vi "SteuerungWaermepumpe.vi"() -> ()   [LabVIEW 2015]
uses:
  <vilib>/DAQmx/read.llb/DAQmx Read (Analog 1D Wfm NChan NSamp).vi
  <vilib>/DAQmx/write.llb/DAQmx Write (Analog 1D Wfm NChan 1Samp).vi
  <vilib>/MakerHub/LINX/Public/Peripherals/Digital/Digital Write N Chans.vi
  <vilib>/DAQmx/miscellaneous.llb/DAQmx Fill In Error Info.vi
  <vilib>/Utility/file.llb/Read Delimited Spreadsheet (DBL).vi
  <vilib>/MakerHub/LINX/LMH-LINX.lvlib
panel:
  out "Abscheider":cluster{dbl, dbl, dbl}(slide) scale=0.0..1.3
  in  "Rampe":bool=TRUE
  in  "Rampe rpm/s":dbl=1.0 min=1.0 max=100.0 step=1.0
  out "Rampe IW":dbl
  in  "reinitialize HD":bool
  in  "reinitialize Pumpe":bool
  out "ist an!":string
  in  "zusätzlicher Druck":dbl
  in  "PI05 SW":dbl format="%.2f"
  out "p_liq_mittel":dbl
  out "p_liq":dbl
  out "Schleifendauer":dbl format="%.5f"
  out "Mittelwert 2":dbl
  in  "Mittelwert HD":bool
  in  "Mittelwert Pumpe":bool
  out "Mittelwert":dbl
  in  "Xi / p_liq berechnung an":bool
  out "xi_r":dbl
  in  "Regler Senke":bool
  in  "reinitialize Senke":bool
  in  "TI35 SW":dbl=43.0 format="%.2f"
  in  "Drehzahl Bestätigung":bool
  in  "Drehzahl SW":dbl=1000.0 min=500.0 max=3000.0 step=1.0 format="%#_4g"
  out "Check":dbl format="%#_13g"
  in  "Regler Hochdruck":bool
  in  "PID Regelung Pumpe":bool
  in  "SW TI39":dbl
  out "Array":bool[](array[boolean])
  in  "LEDs 2":bool[](array[boolean])
  in  "Regelung HK":bool
  in  "zu":bool
  in  "auf":bool
  out "FI_Oel":dbl
  in  "RV 33":dbl(slide) scale=-1.0..1.0
  in  "tag":string
  out "Pumpenwerte":dbl[](array[numeric]) format="%.2f"
  out "Speichert!":bool
  out "Historie":string
  in  "Kommentar":string
  out "refnum out":refnum<file>
  in  "Identität!":string(combo)
  in  "Zeit X in Minuten":dbl(slide)=5.0 min=0.0 max=15.0 scale=5.0..15.0
  out "TI 21a Warnungen":dbl
  out "Leistung":dynamicdata(graph)
  out "TI 37":dbl
  in  "Programm stoppen!":bool
  out "%":sgl(slide) scale=0.0..100.0
  out "kalt":bool
  out "warm":bool
  out "?":T1(array[cluster]) {"?" format="%#.4g"; "Konzentration_reich" format="%#.4g"}
  in  "Mit EES vergleichen":bool
  in  "FI13 SW in l/min":dbl=3.0 min=3.0 max=12.0 step=0.10000000149011612
  out "COP_Oel":dbl
  out "Q-Oel kW":dbl format="%_4g"
  in  "Dateiname!":string
  in  "Comment":bool
  in  "Speichern":bool caption="Aktivieren"
  out "ZU     Ventilstellung 33     AUF":dbl(slide) scale=0.0..100.0 scale format="%.2f"
  in  "Regelventil 34":dbl(slide) min=0.0 max=100.0 step=0.009999999776482582 scale=0.0..100.0
  in  "Matlab":bool
  in  "?":T2(tab)
  out "?":dynamicdata(graph)
  out "?":waveform(dbl)(graph)
  out "?":dynamicdata(graph)
  out "PI 12":dbl format="%.2f"
  out "PI 11":dbl format="%.2f"
  out "Dichte":dbl format="%.5g"
  in  "Reset":bool
  out "Betriebszeit":cluster{"second":i32, "minute":i32, "hour":i32}
  out "Temperatur Ölprüfstand":dbl
  out "FI 13 kg/min":dbl
  in  "Messung\nFrequenzwandler":bool
  out "Magnetventil":bool
  out "Fl.Pumpe an":bool
  out "Temperatur Öl":bool
  out "COP":dbl format="%#_13g"
  out "Verdichteraktivität":cluster{"second":i32, "minute":i32, "hour":i32}
  out "Q-Entgaser kW":dbl format="%_4g"
  out "Warnungen":bool[](array[boolean])
  out "Status Komponenten":bool[](array[boolean])
  in  "Pumpen-Auto-Abschalt":bool=TRUE
  out "Q-Resorber kW":dbl format="%_4g"
  out "Stellung Expansionsventil":waveform(dbl)(graph)
  out "FI 35 l/min":dbl format="%#_13g"
  out "FI 38 l/min":dbl format="%#_13g"
  out "FI Oel l/min":dbl format="%#.3g"
  out "LI in l":dbl format="%#_4g"
  out "TI 39":dbl format="%#_3g"
  out "TI 38":dbl format="%#_3g"
  out "TI 36":dbl format="%#_3g"
  out "TI 35":dbl format="%#_3g"
  out "TI 33":dbl format="%#_3g"
  out "TI 32":dbl format="%#_3g"
  out "TI 34":dbl format="%#_3g"
  out "TI 21a":dbl format="%#_3g"
  out "TI 21":dbl format="%#_3g"
  out "TI 20":dbl format="%#_3g"
  out "TI 14a":dbl format="%#_3g"
  out "TI 14":dbl format="%#_3g"
  out "TI 13":dbl format="%#_3g"
  out "TI 12":dbl format="%#_3g"
  out "TI 11":dbl format="%#_3g"
  out "TI 10":dbl format="%#_3g"
  out "TI 09":dbl format="%#_3g"
  out "TI 08":dbl format="%#_3g"
  out "TI 07":dbl format="%#_3g"
  out "TI 06a":dbl format="%#_3g"
  out "TI 06":dbl format="%#_3g"
  out "TI 05":dbl format="%#_3g"
  out "TI 04":dbl format="%#_3g"
  out "TI 22":dbl format="%#_3g"
  out "TI 02":dbl format="%#_3g"
  out "TI 01":dbl format="%#_3g"
  out "Konzentration":dbl format="%#_5g"
  in  "Pumpensteuerung":dbl min=0.0 max=10.0 step=0.009999999776482582 format="%.2g"
  out "PI 08":dbl format="%.2f"
  out "PI 05":dbl format="%#.2f"
  out "PI 02":dbl format="%.2f"
  out "PI 04":dbl format="%.2f"
  out "PDI 8-9":dbl format="%.2f"
  out "PI 14":dbl format="%.2f"
  out "PI 01":dbl format="%.2f"
  out "ZU    Ventilstellung Exp.V     AUF":dbl(slide) scale=0.0..100.0 scale format="%#.1f"
  in  "Exp.V":dbl(slide)=3.0 min=0.0 max=100.0 step=1.0 scale=0.0..100.0 scale format="%#.0f"
  out "ZU    Ventilstellung 14      AUF":dbl(slide) caption="Auf    Ventilstellung 14      Zu" scale=0.0..100.0 scale format="%#.2f"
  in  "Regelventil 36":dbl(slide) min=0.0 max=100.0 step=0.009999999776482582 scale=0.0..100.0 scale format="%#.0f"
  out "ZU  Ventilstellung 35  AUF":dbl(slide) scale=0.0..100.0 scale format="%.2f"
  in  "Regelventil 35":dbl(slide)=100.0 min=0.0 max=100.0 step=0.009999999776482582 scale=0.0..100.0 scale format="%#.3g"
  out "ZU     Ventilstellung 39     AUF":dbl(slide) scale=0.0..100.0 scale format="%.2f"
  in  "Regelventil 39":dbl(slide)=100.0 min=0.0 max=100.0 step=0.009999999776482582 scale=0.0..100.0
  out "FI 13 l/min":dbl format="%.2f"
  out "FI 07 l/min":dbl format="%.2f"
  out "LI in m":dbl format="%.2f"
  out "PDI 5-6":dbl format="%.4f"
  out "PI 07":dbl format="%.2f"
  out "Druckverhältnis":dbl
  out "Drehzahl":dbl
  out "Drehmoment":dbl
  out "Frequenz":dbl
  out "Leistung":dbl
  out "Durchfluss":waveform(dbl)[](graph)
  in  "Tab Control Temperaturen":T3(tab)
  out "Temperatur Reich":waveform(dbl)[](graph)
  out "Temperatur Arm":waveform(dbl)[](graph)
  out "Temperatur Öl":waveform(dbl)[](graph)
  out "Temperatur Senke/Quelle":waveform(dbl)[](graph)
  out "Druck":waveform(dbl)[](graph)
  out "Druckzustand":bool caption="Zu viel Druck !!!"
  # "Öltemperatur"
  # "Resorber"
  # "Entgaser"
  # "Druckverhältnis"
  # "ExpV"
  # "Verdichter an"
  # "iWÜ"
  # "Magnetventil"
  # "RV 39"
  # "RV 35"
  # "RV 33"
  # "RV 34"
  # "Pumpe an"
  # "Ölabscheider"
  # "2"
  # "1"
  # "RV 30"
  # "Verdichter"
  # "Pumpe"
  # "Leistung"
  # "kW"
  # "Speed"
  # "rpm"
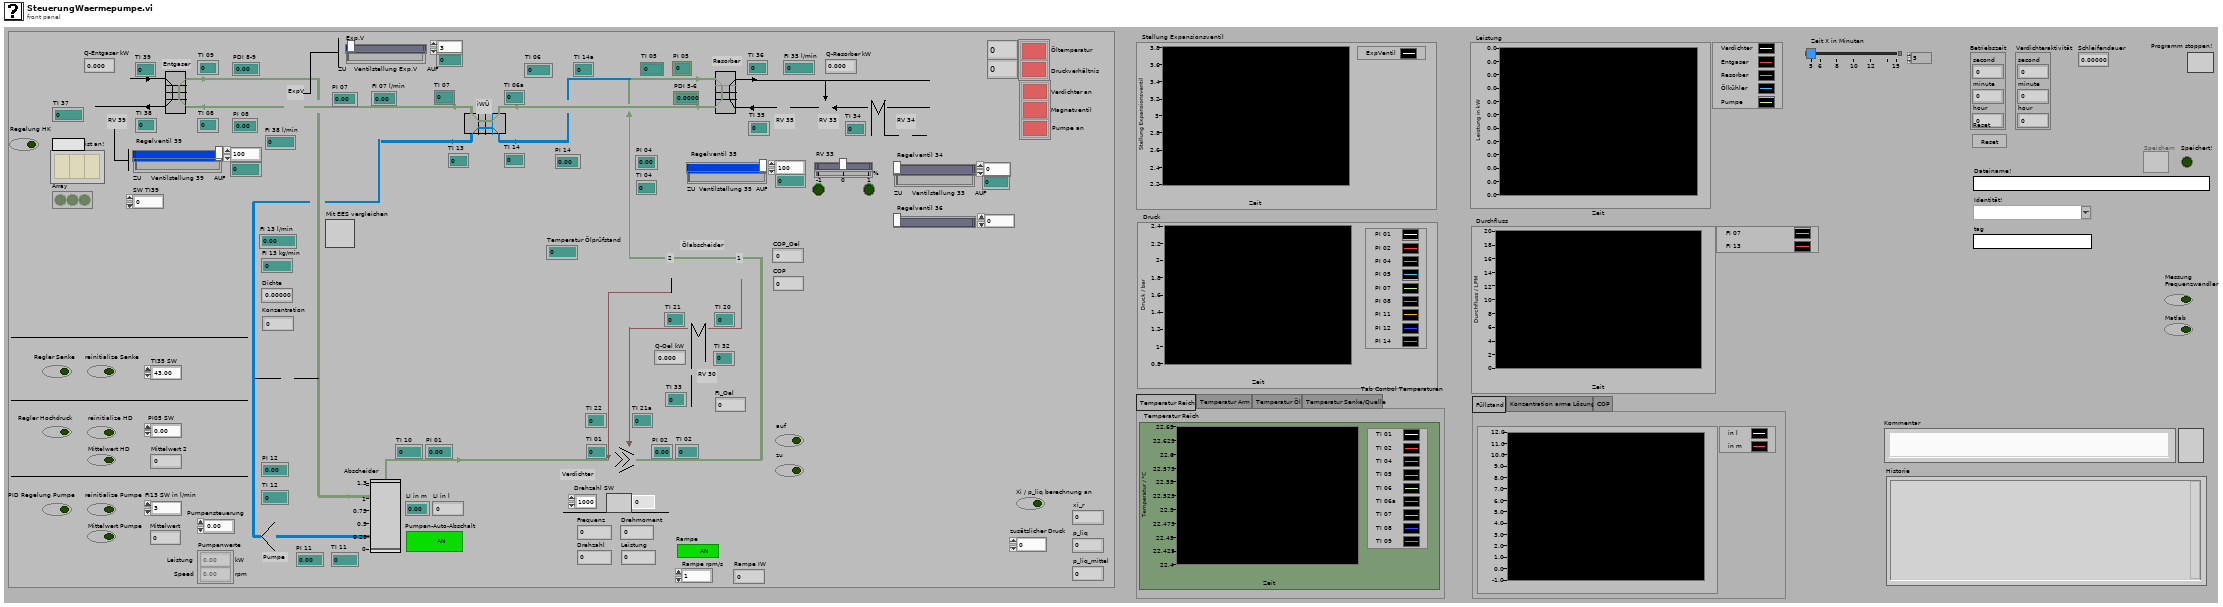
[diagram p1: front panel]
types:
  T1 = cluster{dbl, "Konzentration_reich":dbl, "String":string, bool}[]
  T2 = enum32{"Füllstand", "Konzentration arme Lösung", "COP"}
  T3 = enum32{"Temperatur Reich", "Temperatur Arm", "Temperatur Öl", "Temperatur Senke/Quelle"}
  T4 = enum8{"Enabled", "Disabled", "Disabled and Grayed Out"}
  T5 = typedef "LMH-LINX.lvlib/LINX Ref.ctl" = cluster{"Platform":T6, "Interface":T7, "LINX Device Config":T8}
  T6 = typedef "LMH-LINX.lvlib/Platform.ctl" = enum16{"LINX", "myRIO"}
  T7 = typedef "LMH-LINX.lvlib/Interface.ctl" = enum16{"Serial", "TCP"}
  T8 = typedef "LMH-LINX.lvlib/Device.lvlib/LINX Device Config.ctl" = cluster{"Interface":T7, "COM Port":refnum<visa-resource-name>, "TCP Configuration":T9, "Device Family":u8, "Device ID":u8, "Device Name":string, "TCP Ref":refnum<k5>, "Channels":T10}
  T9 = typedef "LMH-LINX.lvlib/Device.lvlib/TCP Config.ctl" = cluster{"IP Address":string, "Port":u16}
  T10 = typedef "LMH-LINX.lvlib/Channels.ctl" = cluster{"DI":u8[], "DO":u8[], "AI":u8[], "AO":u8[], "PWM":u8[], "QE":u8[], "UART":u8[], "I2C 2":u8[], "SPI":u8[], "CAN":u8[], "Servo":u8[], "AI Ref (V)":dbl, "AO Ref (V)":dbl, "AO Resolution (Bits)":u8}
  T11 = enum16{"open", "replace", "create", "open or create", "replace or create", "replace or create with confirmation"}
  T12 = cluster{"Array[0]":dbl, "Array[1]":dbl, "Array[2]":dbl}
  T13 = cluster{"Array[0]":sgl, "Array[1]":sgl, "Array[2]":sgl}
  T14 = cluster{"Numeric":dbl, "Konzentration_reich":dbl, "String":string, bool}[]
  T15 = typedef "LVDateTimeRec.ctl" = cluster{"fractional second":dbl, "second":i32, "minute":i32, "hour":i32, "day of month":i32, "month":i32, "year":i32, "day of week":i32, "day of year":i32, "DST":i32}
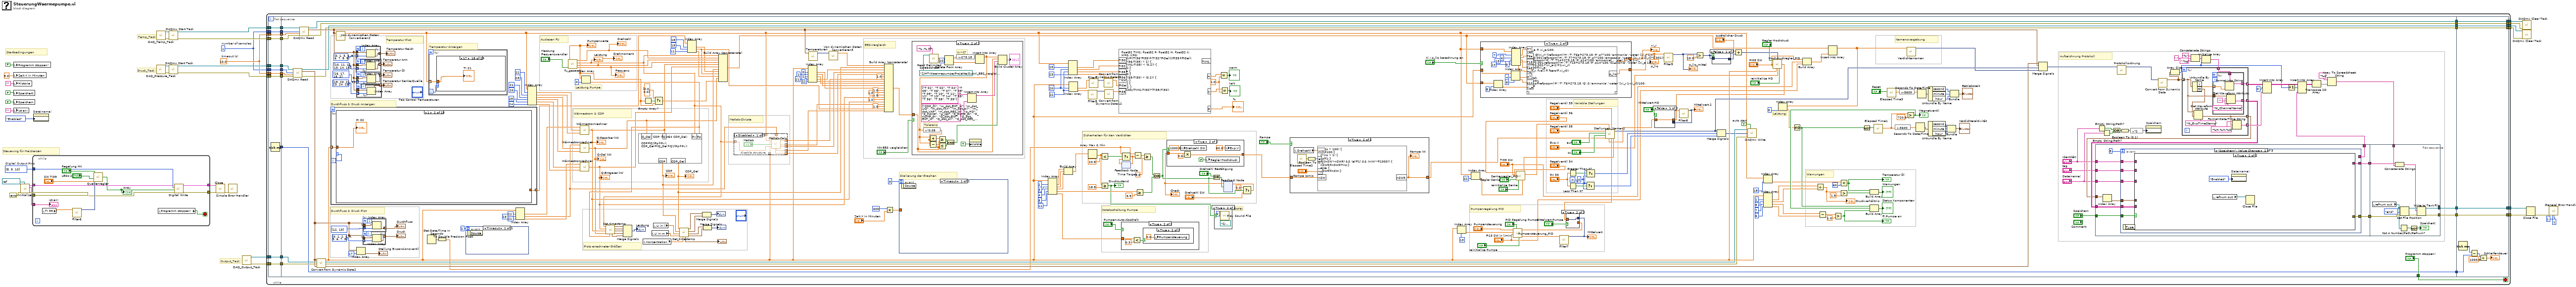
[diagram p0: block diagram]
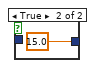
[diagram p5: hidden frame]
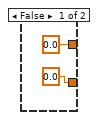
[diagram p8: hidden frame]
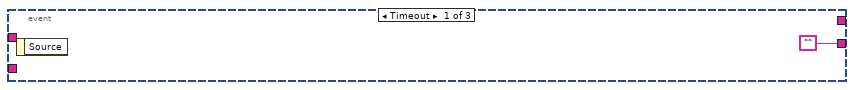
[diagram p10: hidden frame]
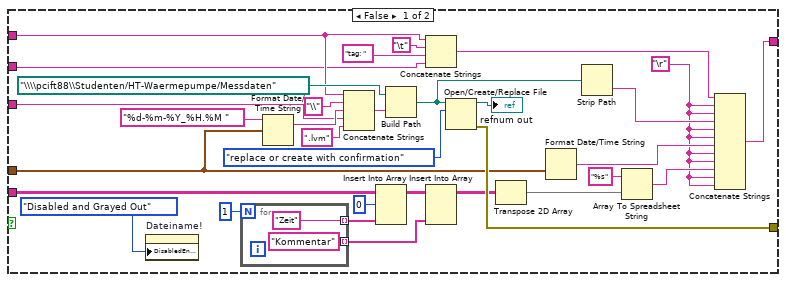
[diagram p11: hidden frame]
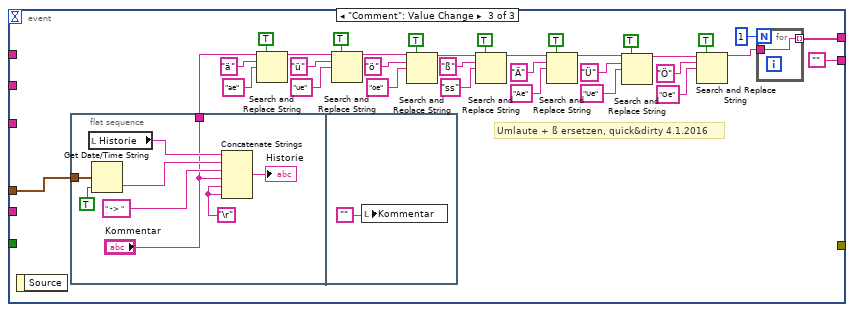
[diagram p12: hidden frame]
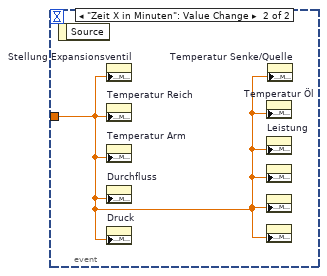
[diagram p13: hidden frame]
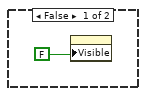
[diagram p14: hidden frame]
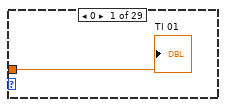
[diagram p17: hidden frame]
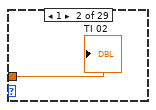
[diagram p18: hidden frame]
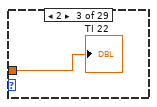
[diagram p19: hidden frame]
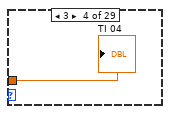
[diagram p20: hidden frame]
diagram:
  w9 = 10.0  # timeout (s)
  w8 = 1  # number of samples
  w21 = i32[] [8, 9, 10]  # Digital Output PIns
  # "Output_Task"
  # "Druck_Task"
  # "Temp_Task"
  # "Steuerung für Heizkerzen"
  # "Startbedingungen"
  n1 = local write "Programm stoppen!"(FALSE ("Programm stoppen!")) -> ()
  n2 = local write "Zeit X in Minuten"(5.0 ("Zeit X in Minuten")) -> ()
  n3 = local write "Historie"("") -> ()
  n4 = local write "Speichert!"(FALSE ("Speichert!")) -> ()
  n5 = local write "Speichern"(FALSE ("Speichern")) -> ()
  n6 = local write "ist an!"("") -> ()
  n7 = call <vilib>:"Initialize.vi"("Serial Port"=refnum<visa-resource-name> "COM3", "Error In"=errorcluster {"status"=FALSE, "code"=0, "source"=""}) -> ("Error Out"=w22:errorcluster, "Device Name"=w19:string, "LINX Ref"=w25:T5)  [unwired: 7 in]
  n8 = while {
    tunnel: w25 -> [w40]
    tunnel: [w50] -> w24
    tunnel: [w49] -> w23
    tunnel: w22 -> [w39]
    tunnel: w21 -> [w48]
    tunnel: w19 -> [w38]
    stop <- w47 stop-if-true
    n9 = local read "TI 39"() -> (w41:dbl)
    n10 = call "Filter6"("Signal"=w41) -> ("Filtered Signal"=w42:dynamicdata)  [unwired: 9 in, 1 out]
    n11 = call "Quellenregler.vi"("Regelung Quelle"="Regelung HK", "TI 38 IW °C"=w42, "LEDs"="LEDs 2", "TI 38 SW °C"="SW TI39") -> ("Kerzen von Regler"=w44:bool[])  [unwired: 3 in, 1 out]
    "Array" <- w44
    n12 = local read "Programm stoppen!"() -> (w47:bool)
    n13 = call-poly <vilib>:"Digital Write.vi"("Error In"=w39, "Values"=w44, "DO Channels"=w48, "LINX Resource"=w40) -> ("Error Out"=w49:errorcluster, "LINX Resource"=w50:T5)  [unwired: 6 in]
    "ist an!" <- w38
  }
  n14 = property on="Dateiname!" class="Str"("DisabledEnum"=T4."Enabled" ("Disabled")) -> ()  [unwired: 2 in, 2 out]
  n15 = call "DAQ_Pressure_Task.vi"() -> ("error out"=w13:errorcluster, "task out"=w14:refnum<k21>)  [unwired: 10 in]
  n16 = call "DAQ_Temp_Task.vi"() -> ("error out"=w15:errorcluster, "task out"=w16:refnum<k21>)  [unwired: 10 in]
  n17 = call <vilib>:"DAQmx Start Task.vi"("task/channels in"=w14, "error in"=w13) -> ("task out"=w7:refnum<k21>, "error out"=w10:errorcluster)  [unwired: 12 in]
  n18 = call <vilib>:"DAQmx Start Task.vi"("task/channels in"=w16, "error in"=w15) -> ("task out"=w11:refnum<k21>, "error out"=w12:errorcluster)  [unwired: 12 in]
  n19 = call <vilib>:"Close.vi"("Error In"=w23, "LINX Resource"=w24) -> ("Error Out"=w26:errorcluster)  [unwired: 8 in, 1 out]
  n20 = call <vilib>:"Simple Error Handler.vi"("error in (no error)"=w26) -> ()  [unwired: 4 in, 5 out]
  n21 = call "DAQ_Output_Task.vi"() -> ("error out"=w1:errorcluster, "task out"=w2:refnum<k21>)  [unwired: 10 in]
  n22 = while {
    tunnel: [w85] -> w31
    tunnel: [w84] -> w30
    tunnel: w12 -> [w78]
    tunnel: w9 -> [w76]
    tunnel: w11 -> [w73]
    tunnel: w8 -> [w71]
    tunnel: w10 -> [w69]
    tunnel: w9 -> [w68]
    tunnel: w8 -> [w66]
    tunnel: w7 -> [w64]
    tunnel: [w60] -> w6
    tunnel: [w59] -> w5
    tunnel: [w57] -> w4
    tunnel: [w55] -> w3
    tunnel: w2 -> [w54]
    tunnel: w1 -> [w51]
    stop <- w83 stop-if-true
    n23 = flat-sequence {
      tunnel: [w96] -> w79
      tunnel: w78 -> [w95]
      tunnel: [w95] -> w77
      tunnel: w76 -> [w94]
      tunnel: [w94] -> w75
      tunnel: w73 -> [w93]
      tunnel: [w93] -> w74
      tunnel: [w92] -> w72
      tunnel: w71 -> [w92]
      tunnel: [w91] -> w70
      tunnel: w69 -> [w91]
      tunnel: w68 -> [w90]
      tunnel: [w90] -> w67
      tunnel: w66 -> [w89]
      tunnel: [w89] -> w65
      tunnel: w64 -> [w88]
      tunnel: [w88] -> w63
      tunnel: w54 -> [w87]
      tunnel: [w87] -> w53
      tunnel: [w86] -> w52
      tunnel: w51 -> [w86]
      tunnel: ["Programm stoppen!"] -> w83
      tunnel: [w304] -> w82
      tunnel: [w303] -> w81
      tunnel: [w102] -> w80
      tunnel: w79 -> [w102]
      tunnel: w77 -> [w143]
      tunnel: w75 -> [w142]
      tunnel: w74 -> [w141]
      tunnel: w72 -> [w140]
      tunnel: w70 -> [w139]
      tunnel: w67 -> [w138]
      tunnel: w65 -> [w137]
      tunnel: w63 -> [w136]
      tunnel: [w135] -> w62
      tunnel: [w134] -> w61
      tunnel: [w133] -> w58
      tunnel: [w132] -> w56
      tunnel: w53 -> [w130]
      tunnel: w52 -> [w129]
      tunnel: [w722] -> w84
      tunnel: [w723] -> w85
      tunnel: w82 -> [w723]
      tunnel: w81 -> [w722]
      tunnel: w80 -> [w720]
      tunnel: w62 -> [w715]
      tunnel: w61 -> [w716]
      tunnel: [w716] -> w60
      tunnel: [w715] -> w59
      tunnel: w58 -> [w714]
      tunnel: [w714] -> w57
      tunnel: w56 -> [w713]
      tunnel: [w713] -> w55
      frame #0 {
        n24 = Tick Count (ms)() -> (millisecond timer value=w96:u32)
      }
      frame #1 {
        w104 = 8.0  # Time Target
        w131 = TRUE  # auto start
        w324 = sgl 1.0
        w337 = 22
        w342 = 20
        w368 = -4
        w369 = 0
        # "ENTE!"
        # "Sicherheiten für den Verdichter"
        # "Pumpenregelung PID"
        # "Skalierung der Graphen"
        # "Leistung Pumpe"
        # "Leistung"
        # "Durchfluss & Druck Anzeigen"
        # "Temperatur Anzeigen"
        # "Plots errechneter Größen"
        # "EES-Vergleich"
        # "Matlab-Skripte"
        # "Warnungen"
        # "Namensvergebung"
        # "Wärmestrom & COP"
        # "Notabschaltung Pumpe"
        # "Auslesen FU"
        # "Durchfluss & Druck Plot"
        # "Temperatur Plot"
        # "Aufzeichnung Protokoll"
        # "Variable Stellungen"
        n25 = call-poly <vilib>:"DAQmx Read.vi"("task/channels in"=w136, "number of samples per channel"=w137, "timeout"=w138, "error in"=w139) -> ("task out"=w135:refnum<k21>, "data"=w145:waveform(dbl)[], "error out"=w132:errorcluster)  [unwired: 9 in]
        n26 = call-poly <vilib>:"DAQmx Read.vi"("task/channels in"=w141, "number of samples per channel"=w140, "timeout"=w142, "error in"=w143) -> ("task out"=w134:refnum<k21>, "data"=w144:waveform(dbl)[], "error out"=w133:errorcluster)  [unwired: 9 in]
        n27 = call "Convert from Dynamic Data2"("Dynamic Data Type"=w145) -> ("Array"=w150:dbl[])  [unwired: 3 in]
        n28 = for {
          tunnel: w150 -> [w661] mode=indexing
          tunnel: [w660] -> w155 mode=indexing
          i -> [w662]
          n29 = case shown="1" w662 {
            tunnel: w661 -> [w663 w664 w665 w666 w667 w668 w669 w670 w671 w672 w673 w682 w694 w697 w698 w699 w700 w701 w704 w708 w709 w710 w711 w712 _]
            tunnel: [_ _ _ _ _ _ _ _ _ _ _ w674 _ _ _ _ _ _ w702 w706 _ _ _ _ _] -> w660
            frame 0 {
              "PI 01" <- w663
            }
            frame 1 {
              "PI 02" <- w664
            }
            frame 2 {
              "PI 04" <- w665
            }
            frame 3 {
              "PI 05" <- w666
            }
            frame 4 {
              "PI 07" <- w667
            }
            frame 5 {
              "PI 08" <- w668
            }
            frame 6 {
              "PI 11" <- w669
            }
            frame 7 {
              "PI 12" <- w670
            }
            frame 8 {
              "PI 14" <- w671
            }
            frame 9 {
              "PDI 5-6" <- w672
            }
            frame 10 {
              "PDI 8-9" <- w673
            }
            frame 11 {
              n30 = call "Filter3"("Signal"=w682) -> ("Filtered Signal"=w680:dynamicdata)  [unwired: 9 in, 1 out]
              n31 = Greater?(x=w682, y=0.3) -> (0:w677:bool)
              n32 = case shown="False" w677 {
                tunnel: w682 -> [_ w693]
                tunnel: [0.0 w693] -> w685
                frame False {
                }
                frame True {
                }
              }
              n33 = call "Convert from Dynamic Data6"("Dynamic Data Type"=w680) -> ("Scalar"=w679:dbl)  [unwired: 3 in]
              n34 = Multiply(x=w679, y=10.0) -> (x*y=w681:dbl)
              n35 = Greater?(x=w682, y=0.4) -> (0:w678:bool)
              n36 = formula code="float64 y; float64 Vu; /*Vu: Volumen schmaler Zylinder+Fuellstandsmesser*/\nVu=10;  /* 10 Liter */\n\nif (x<=10.25) \ny=(x-1)*pi*(0.536**2+0.32**2);\nelse\ny=Vu+(x-10.25)*pi*(1.584**2+0.32**2);"("x"=w681) -> ("y"=w674:dbl)
              "LI in l" <- w674
              n37 = case shown="False" w678 {
                tunnel: w682 -> [_ w691]
                tunnel: [0.0 w691] -> w684
                frame False {
                }
                frame True {
                }
              }
              n38 = Merge Signals(w682, w685, w684) -> (w686:dynamicdata)
              n39 = call "Convert from Dynamic Data3"("Dynamic Data Type"=w686) -> ("Array"=w689:dbl[])  [unwired: 3 in]
              n40 = Array To Cluster(array=w689) -> (cluster=w676:T12)
              n41 = To Single Precision Float(number=w676) -> (single precision float=→"Abscheider":T13)
              "LI in m" <- w682
            }
            frame 12 {
              "FI 07 l/min" <- w694
            }
            frame 13 {
              n42 = local read "Dichte"() -> (w696:dbl)
              n43 = Multiply(x=w697, y=w696) -> (x*y=→"FI 13 kg/min":dbl)
              "FI 13 l/min" <- w697
            }
            frame 14 {
              "ZU     Ventilstellung 39     AUF" <- w698
              "ZU     Ventilstellung 33     AUF" <- w698
            }
            frame 15 {
              "ZU  Ventilstellung 35  AUF" <- w699
            }
            frame 16 {
              # "RV14 ist entfernt"
              "ZU    Ventilstellung 14      AUF" <- w700
            }
            frame 17 {
              "ZU    Ventilstellung Exp.V     AUF" <- w701
            }
            frame 18 {
              n44 = call "Filter"("Signal"=w704) -> ("Filtered Signal"=w703:dynamicdata)  [unwired: 9 in, 1 out]
              n45 = call "Convert from Dynamic Data4"("Dynamic Data Type"=w703) -> ("Scalar"=w705:dbl)  [unwired: 3 in]
              n46 = formula code="float64 D;\nD=9.375*StromDichte+0.7125;\nD=floor(D*100000)/100000;"("StromDichte"=w705) -> ("D"=w702:dbl)
              "Dichte" <- w702
            }
            frame 19 {
              n47 = call "Filter2"("Signal"=w708) -> ("Filtered Signal"=w707:dynamicdata)  [unwired: 9 in, 1 out]
              n48 = To Double Precision Float(number=w707) -> (double precision float=w706:dbl)
              "Konzentration" <- w706
            }
            frame 20 {
              "FI Oel l/min" <- w709
            }
            frame 21 {
              "FI 38 l/min" <- w710
            }
            frame 22 {
              "FI 35 l/min" <- w711
            }
            frame 23 {
              "FI_Oel" <- w712
            }
            frame 24, Default {
            }
          }
        }
        n49 = call "Von dynamischen Daten konvertieren2"("Dynamic Data Type"=w144) -> ("Array"=w125:dbl[])  [unwired: 3 in]
        n50 = for {
          tunnel: i32[] [0, 1, 3, 4, 5, 6, 7, 8, 9] -> [w475] mode=indexing
          tunnel: w144 -> [w474]
          tunnel: [w473] -> w240 mode=indexing
          n51 = Index Array(array=w474, index=w475) -> (element=w473:waveform(dbl))
        }
        "Temperatur Reich" <- w240
        n52 = for {
          tunnel: i32[] [10, 11, 12, 13, 14, 15] -> [w472] mode=indexing
          tunnel: w144 -> [w471]
          tunnel: [w470] -> w241 mode=indexing
          n53 = Index Array(array=w471, index=w472) -> (element=w470:waveform(dbl))
        }
        "Temperatur Arm" <- w241
        n54 = for {
          tunnel: i32[] [16, 17, 18, 2] -> [w469] mode=indexing
          tunnel: w144 -> [w468]
          tunnel: [w467] -> w242 mode=indexing
          n55 = Index Array(array=w468, index=w469) -> (element=w467:waveform(dbl))
        }
        "Temperatur Öl" <- w242
        n56 = Index Array(array=w145, index=17) -> (element=→"Stellung Expansionsventil":waveform(dbl))
        n57 = for {
          tunnel: i32[] [19, 20, 21, 22, 23, 24, 25] -> [w466] mode=indexing
          tunnel: w144 -> [w465]
          tunnel: [w464] -> w243 mode=indexing
          n58 = Index Array(array=w465, index=w466) -> (element=w464:waveform(dbl))
        }
        "Temperatur Senke/Quelle" <- w243
        n59 = for {
          tunnel: [w460] -> w238 mode=indexing
          tunnel: w145 -> [w459]
          tunnel: i32[] [0, 1, 2, 3, 4, 5, 6, 7, 8] -> [w458] mode=indexing
          n60 = Index Array(array=w459, index=w458) -> (element=w460:waveform(dbl))
        }
        "Druck" <- w238
        n61 = for {
          tunnel: [w463] -> w239 mode=indexing
          tunnel: w145 -> [w462]
          tunnel: i32[] [12, 13] -> [w461] mode=indexing
          n62 = Index Array(array=w462, index=w461) -> (element=w463:waveform(dbl))
        }
        "Durchfluss" <- w239
        n63 = Get Date/Time In Seconds() -> (seconds since 1Jan1904=w101:timestamp)
        n64 = for {
          tunnel: w125 -> [w630] mode=indexing
          i -> [w631]
          n65 = case shown="17" w631 {
            tunnel: w630 -> [w632 w633 w634 w635 w636 w637 w638 w639 w640 w641 w642 w643 w644 w645 w646 w647 w648 w649 w650 w651 w652 w653 w654 w655 w656 w657 w658 w659 _]
            frame 0 {
              "TI 01" <- w632
            }
            frame 1 {
              "TI 02" <- w633
            }
            frame 2 {
              "TI 22" <- w634
            }
            frame 3 {
              "TI 04" <- w635
            }
            frame 4 {
              "TI 05" <- w636
            }
            frame 5 {
              "TI 06" <- w637
            }
            frame 6 {
              "TI 06a" <- w638
            }
            frame 7 {
              "TI 07" <- w639
            }
            frame 8 {
              "TI 08" <- w640
            }
            frame 9 {
              "TI 09" <- w641
            }
            frame 10 {
              "TI 10" <- w642
            }
            frame 11 {
              "TI 11" <- w643
            }
            frame 12 {
              "TI 12" <- w644
            }
            frame 13 {
              "TI 13" <- w645
            }
            frame 14 {
              "TI 14" <- w646
            }
            frame 15 {
              "TI 14a" <- w647
            }
            frame 16 {
              "TI 20" <- w648
            }
            frame 17 {
              "TI 21" <- w649
            }
            frame 18 {
              "TI 21a" <- w650
              "TI 21a Warnungen" <- w650
            }
            frame 19 {
              # "Check T_Heater"
              "TI 34" <- w651
            }
            frame 20 {
              "TI 32" <- w652
            }
            frame 21 {
              "TI 33" <- w653
            }
            frame 22 {
              "TI 35" <- w654
            }
            frame 23 {
              "TI 36" <- w655
            }
            frame 24 {
              "TI 38" <- w656
            }
            frame 25 {
              "TI 39" <- w657
            }
            frame 26 {
              "Temperatur Ölprüfstand" <- w658
            }
            frame 27 {
              "TI 37" <- w659
            }
            frame 28, Default {
            }
          }
        }
        n66 = To Double Precision Float(number=w101) -> (double precision float=w100:dbl)
        n67 = event shown="[0] Timeout" {
          selector: _ -> [_]
          dyn-events: _ -> [_]
          timeout: 2 -> [_]
          event Timeout {
            n68 = event-data() -> ()  [unwired: 1 in, 1 out]
          }
        }
        n69 = Index Array(array=w150, index #1=22 ("index"), index #2=23 ("index"), index #3=21 ("index")) -> (element #1=w273:dbl, element #2=w249:dbl, element #3=w272:dbl)
        n70 = Index Array(array=w125, index #1=22 ("index"), index #2=23 ("index"), index #3=21 ("index"), index #4=20 ("index"), index #5=25 ("index"), index #6=24 ("index")) -> (element #1=w271:dbl, element #2=w270:dbl, element #3=w269:dbl, element #4=w268:dbl, element #5=w267:dbl, element #6=w266:dbl)
        n71 = call "fu_gesamt.vi"("Boolean"="Messung\nFrequenzwandler") -> ("Frequenz"=w261:dbl, "Drehmoment"=w262:dbl, "Leistung"=w113:dbl, "Drehzahl"=w263:dbl, "Scaled"=w115:dbl[])  [unwired: 6 in]
        "Leistung" <- w113
        "Frequenz" <- w261
        "Drehmoment" <- w262
        "Drehzahl" <- w263
        "Pumpenwerte" <- w115
        n72 = call "Wärmestromrechner.vi"("Taus"=w270, "Tein"=w271, "Massenstrom"=w273) -> ("Wärmestrom Q"=w169:dbl)  [unwired: 2 in]
        "Q-Resorber kW" <- w169
        n73 = call "Wärmestromrechner.vi"("Taus"=w268, "Tein"=w269, "Massenstrom"=w249) -> ("Wärmestrom Q"=w156:dbl)  [unwired: 2 in]
        "Q-Oel kW" <- w156
        n74 = call "Wärmestromrechner.vi"("Taus"=w266, "Tein"=w267, "Massenstrom"=w272) -> ("Wärmestrom Q"=w168:dbl)  [unwired: 2 in]
        "Q-Entgaser kW" <- w168
        n75 = Index Array(array=w115, index=0) -> (element=w170:dbl)
        n76 = call "Set_timestamp.vi"("Eingang 5"=w170, "Eingang 4"=w156, "Eingang 3"=w169, "Eingang 2"=w168, "Eingang"=w113) -> ("Ausgang 4"=w166:waveform(dbl), "Ausgang 3"=w165:waveform(dbl), "Ausgang 2"=w164:waveform(dbl), "Ausgang"=w163:waveform(dbl), "Ausgang 5"=w167:waveform(dbl))  [unwired: 2 in]
        n77 = Merge Signals(w163, w164, w165, w166, w167) -> (→"Leistung":dynamicdata)
        n78 = formula code="float64 COP; float64 COP_Oel;\n\nCOP=Q/(Pp+Pv);\nCOP_Oel=(Q_Oel+Q)/(Pp+Pv);"("Pv"=w113, "Q"=w169, "Pp"=w170, "Q_Oel"=w156) -> ("COP"=w178:dbl, "COP_Oel"=w177:dbl)
        "COP" <- w178
        "COP_Oel" <- w177
        n79 = local read "Konzentration"() -> (w182:dbl)
        n80 = Empty Array?(array=w115) -> (empty?=w117:bool)
        n81 = local read "LI in m"() -> (w180:dbl)
        n82 = local read "LI in l"() -> (w179:dbl)
        n83 = Select(t=dbl[] [0.0, 0.0], s=w117, f=w115) -> (s? t:f=w114:dbl[])
        n84 = call "Set_timestamp.vi"("Eingang 5"=w182, "Eingang 4"=w180, "Eingang 3"=w179, "Eingang 2"=w178, "Eingang"=w177) -> ("Ausgang 4"=w175:waveform(dbl), "Ausgang 3"=w174:waveform(dbl), "Ausgang 2"=w172:waveform(dbl), "Ausgang"=w171:waveform(dbl), "Ausgang 5"=→"?":waveform(dbl))  [unwired: 2 in]
        n85 = Index Array(array=w155, index #1=18 ("index"), index #2=19 ("index"), index #3=11 ("index")) -> (element #1=w157:dbl, element #2=w154:dbl, element #3=w158:dbl)
        n86 = Merge Signals(w171, w172) -> (→"?":dynamicdata)
        n87 = Merge Signals(w174, w175) -> (→"?":dynamicdata)
        n88 = Build Array (concatenate)(w113, w263, w262, w261, w169, w168, w178, w157, w154, w158, w156, w114) -> (w120:dbl[])
        n89 = disable-structure shown="Disabled" {
          disable-tunnel: [w420 _] -> w365
          disable-tunnel: [w419 _] -> w354
          disable-tunnel: [w418 _] -> w343
          disable-tunnel: [w417 _] -> w265
          disable-tunnel: [w416 _] -> w260
          disable-tunnel: w249 -> [w415 _]
          disable-tunnel: w113 -> [w414 _]
          disable-tunnel: w150 -> [w413 _]
          disable-tunnel: w125 -> [w412 _]
          frame Disabled {
            n90 = call "Matlab-Calc.vi"("Temp-Array"=w412, "Matlab?"="Matlab", "Leistung"=w414, "Druck-Array"=w413, "FI Öl"=w415) -> ("m_reich [g/s]"=w419:dbl, "Konzentration_reich"=w416:dbl, "m_arm [g/s]"=w420:dbl, "Dampfmassenstrom [g/s]"=w417:dbl, "Dampfmassenanteil"=w418:dbl)  [unwired: 3 in, 7 out]
          }
          frame Enabled {
          }
        }
        n91 = Index Array(array=w150, index #1=0 ("index"), index #2=1 ("index"), index #3=2 ("index"), index #4=21 ("index"), index #5=22 ("index")) -> (element #1=w348:dbl, element #2=w349:dbl, element #3=w350:dbl, element #4=w347:dbl, element #5=w345:dbl)
        n92 = call "Temperaturen"("Signals"=w144) -> ("Signal Out"=w355:dynamicdata)  [unwired: 9 in, 1 out]
        n93 = call "Von dynamischen Daten konvertieren3"("Dynamic Data Type"=w355) -> ("Array"=w356:dbl[])  [unwired: 3 in]
        n94 = Build Array (concatenate)(w356, w177, w347, w365, w354, 1.0 ("element"), w265, w345, w350, w349, w348, 1.0 ("element"), 1.0 ("element"), 1.0 ("element"), w168, 1.0 ("element"), w169, w343, 1.0 ("element"), w154, w260) -> (w357:dbl[])
        n95 = Multiply(x=600, y="Zeit X in Minuten") -> (x*y=w316:dbl)
        n96 = event shown="[0] Timeout" {
          selector: _ -> [_ _]
          dyn-events: _ -> [_ _]
          timeout: 5 -> [_ _]
          tunnel: w316 -> [_ w604]
          event Timeout {
            n97 = event-data() -> ()  [unwired: 1 in, 1 out]
          }
          event "Zeit X in Minuten": Value Change {
            n98 = event-data() -> ()  [unwired: 1 in, 1 out]
            n99 = property on="Stellung Expansionsventil" class="WFChart (strict)"("XScale.Maximum"=w604) -> ()  [unwired: 2 in, 2 out]
            n100 = property on="Temperatur Reich" class="WFChart (strict)"("XScale.Maximum"=w604) -> ()  [unwired: 2 in, 2 out]
            n101 = property on="Temperatur Arm" class="WFChart (strict)"("XScale.Maximum"=w604) -> ()  [unwired: 2 in, 2 out]
            n102 = property on="Durchfluss" class="WFChart (strict)"("XScale.Maximum"=w604) -> ()  [unwired: 2 in, 2 out]
            n103 = property on="Druck" class="WFChart (strict)"("XScale.Maximum"=w604) -> ()  [unwired: 2 in, 2 out]
            n104 = property on="Temperatur Öl" class="WFChart (strict)"("XScale.Maximum"=w604) -> ()  [unwired: 2 in, 2 out]
            n105 = property on="Leistung" class="WFChart (strict)"("XScale.Maximum"=w604) -> ()  [unwired: 2 in, 2 out]
            n106 = property class="WFChart (strict)"("XScale.Maximum"=w604) -> ()  [unwired: 2 in, 2 out]
            n107 = property class="WFChart (strict)"("XScale.Maximum"=w604) -> ()  [unwired: 2 in, 2 out]
            n108 = property class="WFChart (strict)"("XScale.Maximum"=w604) -> ()  [unwired: 2 in, 2 out]
            n109 = property on="Temperatur Senke/Quelle" class="WFChart (strict)"("XScale.Maximum"=w604) -> ()  [unwired: 2 in, 2 out]
          }
        }
        n110 = case shown="True" "Mit EES vergleichen" {
          tunnel: w357 -> [_ w606]
          frame False {
            n111 = property class="Arr (strict)"("Visible"=FALSE) -> ()  [unwired: 2 in, 2 out]
          }
          frame True {
            # "K->C°"
            # "Toleranz"
            n112 = call-poly <vilib>:"Read Delimited Spreadsheet.vi"("file path (dialog if empty)"=path "Z:/HT-Waermepumpe/Projekte/SubVi_EES_vergleich/test.txt", "format (%.3f)"="%,;%.3f") -> ("first row"=w613:dbl[])  [unwired: 8 in, 5 out]
            n113 = Delete From Array(array=w613, length=20) -> (deleted portion=w609:dbl[], array with subset deleted=w611:dbl[])  [unwired: 1 in]
            n114 = expression code="x-273.15"(w611) -> (w610:dbl[])
            n115 = Insert Into Array(array=string[] ["T 01", "T 02", "T 04", "T 05", "T 06", "T 07", "T 08", "T 09", "T 10", "T 11", "T 12", "T 13", "T 14", "T 35", "T 36", "T 38", "T 39"] ("Array"), new element=string[] ["COP_Öl", "m_dot_ENT_W", "m_dot_LIQ", "m_dot_MIX", "m_dot_oil", "m_dot_VAP", "m_dot_RES_W", "p_HD", "P_KOMP", "p_ND", "P_PUMP_th", "P_KOMP_th", "Q_dot_ENT", "Q_dot_ENT_W", "Q_dot_oil", "Q_dot_RES_W", "q_geg", "Q_dot_RES", "xi_LIQ", "xi_MIX"] ("Array")) -> (w620:string[])  [unwired: 1 in]
            n116 = property class="Arr (strict)"("Visible"=TRUE) -> ()  [unwired: 2 in, 2 out]
            n117 = Insert Into Array(array=w610, new element=w609) -> (w607:dbl[])  [unwired: 1 in]
            n118 = expression code="x*0.05"(w607) -> (w608:dbl[])
            n119 = Add(x=w607, y=w608) -> (x+y=w616:dbl[])
            n120 = Subtract(x=w607, y=w608) -> (x-y=w615:dbl[])
            n121 = Greater Or Equal?(x=w616, y=w606) -> (x >= y?=w617:bool[])
            n122 = Less Or Equal?(x=w615, y=w606) -> (x <= y?=w618:bool[])
            n123 = And(x=w617, y=w618) -> (x .and. y?=w614:bool[])
            n124 = Build Cluster Array(w607, w606, w620, w614) -> (→"?":T14)
          }
        }
        n125 = Index Array(array=w150, index #1=2 ("index"), index #2=3 ("index"), index #3=4, index #4=5, index #5=11 ("index")) -> (element #1=w219:dbl, element #2=w218:dbl, element #3=w217:dbl, element #4=w223:dbl, element #5=w199:dbl)
        n126 = Build Array(w219, w218, w217) -> (w216:dbl[])
        n127 = Index Array(array=w125, index #1=19, index #2=w342, index #3=w337, index #4=23) -> (element #1=w334:dbl, element #2=w333:dbl, element #3=w332:dbl, element #4=w331:dbl)
        n128 = Index Array(array=w150, index #1=w342, index #2=w337) -> (element #1=w340:dbl, element #2=w339:dbl)
        n129 = Array Max & Min(array=w216) -> (min value=w108:dbl)  [unwired: 3 out]
        n130 = call "Filter5"("Signal"=w339) -> ("Filtered Signal"=w335:dynamicdata)  [unwired: 9 in, 1 out]
        n131 = call "Filter4"("Signal"=w340) -> ("Filtered Signal"=w336:dynamicdata)  [unwired: 9 in, 1 out]
        n132 = Less?(x=w108, y=20.5 ("x")) -> (x < y?=w106:bool)
        n133 = Greater Or Equal?(x=w108, y=18.5 ("x")) -> (x >= y?=w107:bool)
        "Druckzustand" <- w107
        n134 = call "Convert from Dynamic Data11"("Dynamic Data Type"=w336) -> ("Scalar"=w330:dbl)  [unwired: 3 in]
        n135 = call "Convert from Dynamic Data12"("Dynamic Data Type"=w335) -> ("Scalar"=w329:dbl)  [unwired: 3 in]
        n136 = formula code="float32 TIM1; float32 P; float32 H; float32 K;\nH=0; K=0;\nTIM1=((TI36*FI35)+(TI32*FIOel))/(FI35+FIOel);\nif((TI36-TI35) > 2) {\nif((TIM1-TI35) < (0.2)) {\nH=1;}\nelse {\nH=0;}\nif((TI35-TI30) < (0.2)) {\nK=1;}\nelse {\nK=0; }\nP=100/(TIM1-TI30)*(TI35-TI30);\n}"("TI30"=w334, "TI32"=w333, "TI35"=w332, "TI36"=w331, "FIOel"=w330, "FI35"=w329) -> ("H"=w328:sgl, "K"=w325:sgl, "P"=→"%":sgl)  [unwired: 1 out]
        n137 = case shown="True" "Pumpen-Auto-Abschalt" {
          tunnel: w199 -> [_ w627]
          frame False {
          }
          frame True {
            n138 = Less?(x=w627, y=0.3) -> (x < y?=w626:bool)
            n139 = case shown="True" w626 {
              frame False {
              }
              frame True {
                n140 = local write "Pumpensteuerung"(0.0) -> ()
              }
            }
          }
        }
        n141 = feedback #1() -> (w97:dbl)  [unwired: 1 in]
        n142 = Select(t=w100, s=w106, f=w97) -> (s? t:f=w98:dbl)
        n143 = feedback-in #1(w98) -> ()
        n144 = Subtract(x=w100, y=w98) -> (x-y=w105:dbl)
        n145 = Greater Or Equal?(x=w223, y=9.9 ("x")) -> (x >= y?=w227:bool)
        n146 = Greater Or Equal?(x=w105, y=w104) -> (x >= y?=w103:bool)
        n147 = Or(x=w103, y=w227) -> (x .or. y?=w209:bool)
        n148 = Or(x="Drehzahl Bestätigung", y=w209) -> (x .or. y?=w211:bool)
        n149 = case shown="True" w107 {
          frame False {
          }
          frame True {
            n150 = call <vilib>:"Play Sound File.vi"("path"=path "C:/Users/Hybrid/Desktop/ente_1.wav", "device ID"=u32 0) -> ()  [unwired: 8 in, 2 out]
          }
        }
        n151 = Equal?(x=w328, y=w324) -> (x = y?=→"warm":bool)
        n152 = Equal?(x=w325, y=w324) -> (x = y?=→"kalt":bool)
        n153 = feedback #2() -> (w210:dbl)  [unwired: 1 in]
        "Check" <- w210
        n154 = case shown="True" w209 {
          tunnel: w210 -> [w451 w455]
          tunnel: [w451 w456] -> w112
          frame False {
          }
          frame True {
            n155 = local write "Drehzahl SW"(1000.0) -> ()
            n156 = Multiply(x=w455, y=0.0) -> (x*y=w456:dbl)
            n157 = local write "Regler Hochdruck"(FALSE ("Regler Hochdruck")) -> ()
            n158 = local write "Exp.V"(60.0 ("Exp.V")) -> ()
          }
        }
        n159 = Select(t=0.0, s=w209, f="Drehzahl SW") -> (s? t:f=w213:dbl)
        n160 = feedback-in #2(w213, w211) -> ()
        n161 = case shown="True" "Rampe" {
          tunnel: [w405 w406] -> w111
          tunnel: w112 -> [w405 w408]
          frame False {
          }
          frame True {
            n162 = local read "Drehzahl"() -> (w407:dbl)
            n163 = call "Elapsed Time2"() -> ("Time has Elapsed"=w410:bool)  [unwired: 12 in, 7 out]
            n164 = Boolean To (0,1)(Boolean=w410) -> (0, 1=w409:i16)
            n165 = formula code="if (ns > 100) {\nns=100;}\nif (ns < 1) {\nns=1;}\nif ((nSW>nSWR) && (el=1) && (nIW>=1000)) {\nnSWR=nSWR+ns;}\nelse {\nnSWR=nSW;}"("nSW"=w408, "ns"="Rampe rpm/s", "el"=w409, "nIW"=w407) -> ("nSWR"=w406:dbl)
            "Rampe IW" <- w406
          }
        }
        n166 = Index Array(array=w150, index=13) -> (element=w152:dbl)
        n167 = Index Array(array=w125, index=22) -> (element=w124:dbl)
        n168 = case shown="True" "Xi / p_liq berechnung an" {
          tunnel: w125 -> [_ w450]
          tunnel: w150 -> [_ w443]
          tunnel: [0.0 w436] -> w201
          tunnel: [0.0 w433] -> w191
          tunnel: w120 -> [_ w430]
          frame False {
          }
          frame True {
            n169 = Index Array(array=w430, index=8) -> (element=w432:dbl)
            n170 = Index Array(array=w443, index #1=4 ("index"), index #2=8 ("index")) -> (element #1=w438:dbl, element #2=w437:dbl)
            n171 = Index Array(array=w450, index #1=7 ("index"), index #2=6 ("index"), index #3=13 ("index"), index #4=14 ("index"), index #5=5 ("index")) -> (element #1=w442:dbl, element #2=w441:dbl, element #3=w440:dbl, element #4=w439:dbl, element #5=w434:dbl)
            n172 = script code="xi_a = xi_a/100;\ntry\nF = @(xi_r) ((refpropm('H','T',T6a+273.15,'P',p7*100,'ammonia','water',[xi_r 1-xi_r])*0.001-refpropm('H','T',T7+273.15,'P',p7*100,'ammonia','water',[xi_r 1-xi_r])*0.001)/(refpropm('H','T',T14+273.15,'P',p14*100,'ammonia','water',[xi_a 1-xi_a])*0.001-refpropm('H','T',T13+273.15,'P',p14*100,'ammonia','water',[xi_a 1-xi_a])*0.001)*(xi_a-1)+1-xi_r);\nxi_r0=xi_a;\n[xi_r, fval] = fzero(F,xi_r0);\n\n\ncatch\nxi_r=1\np_liq=refpropm('P','T',T6+273.15,'Q',0,'ammonia','water',[xi_r 1-xi_r])/100;\nend"("T7"=w442, "T6a"=w441, "T13"=w440, "T14"=w439, "xi_a"=w432, "p7"=w438, "p14"=w437, "T6"=w434) -> ("xi_r"=w436:dbl, "p_liq"=w433:dbl)  [unwired: 1 in, 1 out]
          }
        }
        "xi_r" <- w201
        "p_liq" <- w191
        n173 = call "Pumpensteuerung_PID.vi"("reinitialize? (F)"="reinitialize Pumpe", "PID Regelung Pumpe"="PID Regelung Pumpe", "FI13 SW in l/min"="FI13 SW in l/min", "Prozessvariable"=w152, "Pumpensteuerung"="Pumpensteuerung") -> ("upper limit"=w196:dbl)  [unwired: 4 in, 2 out]
        n174 = call "Senkenregler_PID.vi"("Regelventil 36"="Regelventil 36", "Solltemp."="TI35 SW", "Regelventil 34"="Regelventil 34", "Regler Senke"="Regler Senke", "reinitialize?"="reinitialize Senke", "Numeric"=w124) -> ("upper limit 2"=w205:dbl, "upper limit"=w203:dbl)  [unwired: 6 in, 2 out]
        n175 = call "Filter7"("Signal"=w196) -> ("Filtered Signal"=w195:dynamicdata)  [unwired: 9 in, 1 out]
        "Mittelwert" <- w195
        n176 = case shown="True" "Mittelwert Pumpe" {
          tunnel: w196 -> [w426 _]
          tunnel: [w426 w427] -> w197
          tunnel: w195 -> [_ w427]
          frame False {
          }
          frame True {
          }
        }
        n177 = Greater Than 0?(x="RV 33") -> (x > 0?=w233:bool)
        n178 = Less Than 0?(x="RV 33") -> (x < 0?=w232:bool)
        n179 = Select(t=w368, s=w232, f=w369) -> (s? t:f=w366:i32)
        n180 = Select(t=w368, s=w233, f=w369) -> (s? t:f=w367:i32)
        n181 = call "Filter9"("Signal"=w191) -> ("Filtered Signal"=w189:dynamicdata)  [unwired: 9 in, 1 out]
        "p_liq_mittel" <- w189
        n182 = Greater?(x=w189, y=15.0) -> (0:w188:dynamicdata)
        n183 = case shown="False" w188 {
          tunnel: [w422 15.0 ("y")] -> w187
          tunnel: w188 -> [w422 _]
          frame False {
          }
          frame True {
          }
        }
        n184 = Add(x="zusätzlicher Druck", y=w187) -> (x+y=w186:dynamicdata)
        n185 = Index Array(array=w125, index=18) -> (element=w256:dbl)
        n186 = Index Array(array=w150, index #1=1, index #2=5, index #3=7, index #4=6) -> (element #1=w253:dbl, element #2=w252:dbl, element #3=w251:dbl, element #4=w250:dbl)
        n187 = call "Hochdruckregler_PID.vi"("Regler Hochdruck"="Regler Hochdruck", "Dynamic Data"=w186, "Solldruck"="PI05 SW", "PI05"=w150, "Exp.V"="Exp.V", "reinitialize? (F) in"="reinitialize HD") -> ("upper limit out"=w127:dbl)  [unwired: 7 in, 2 out]
        n188 = call "Filter8"("Signal"=w127) -> ("Filtered Signal"=w192:dynamicdata)  [unwired: 9 in, 1 out]
        "Mittelwert 2" <- w192
        n189 = case shown="False" "Mittelwert HD" {
          tunnel: w127 -> [w424 _]
          tunnel: [w424 w425] -> w193
          tunnel: w192 -> [_ w425]
          frame False {
          }
          frame True {
          }
        }
        n190 = call "Stellungen_Namen2.vi"("Kühlventil"=w205, "Pumpensteuerung"=w197, "Regelventil 39"="Regelventil 39", "Exp.V"=w193, "Regelventil 14"=w203, "Meter"=w111, "zu"="zu", "auf"="auf", "Regelventil 35"="Regelventil 35") -> ("Dynamic Data"=w264:dynamicdata)  [unwired: 2 in]
        n191 = Merge Signals(w264, w367, w366) -> (w128:dynamicdata)
        n192 = call-poly <vilib>:"DAQmx Write.vi"("task/channels in"=w130, "auto start"=w131, "data"=w128, "error in"=w129) -> ()  [unwired: 9 in, 3 out]
        n193 = Build Array("PI05 SW", "TI35 SW", "FI13 SW in l/min") -> (w118:dbl[])
        n194 = Divide(x=w253, y=w252) -> (x/y=w374:dbl)
        "Druckverhältnis" <- w374
        n195 = Subtract(x=w251, y=w250) -> (x-y=w386:dbl)
        n196 = Insert Into Array(array=w120, new element=w118) -> (w119:dbl[])  [unwired: 1 in]
        n197 = Index Array(array=w119, index=0) -> (element=w183:dbl)
        n198 = Not Equal To 0?(x=w183) -> (x != 0?=w184:bool)
        n199 = Greater?(x=w386, y=1.0) -> (0:w258:bool)
        "Fl.Pumpe an" <- w258
        n200 = Less?(x=w256, y=60) -> (x < y?=w320:bool)
        "Temperatur Öl" <- w320
        n201 = Greater?(x=w374, y=1.5) -> (0:w372:bool)
        n202 = Not(x=w184) -> (.not. x?=w394:bool)
        n203 = Build Array(w320, w372) -> (→"Warnungen":bool[])
        n204 = call "Elapsed Time1"("Reset"=w394) -> ("Elapsed Time (s)"=w378:dbl)  [unwired: 11 in, 7 out]
        n205 = call "Elapsed Time3"("Reset"="Reset") -> ("Elapsed Time (s)"=w380:dbl)  [unwired: 11 in, 7 out]
        n206 = expression code="x-3600"(w378) -> (w377:dbl)
        n207 = expression code="x-3600"(w380) -> (w381:dbl)
        n208 = Greater?(x=w378, y=720.0) -> (0:w259:bool)
        "Magnetventil" <- w259
        n209 = Build Array(w184, w259, w258) -> (→"Status Komponenten":bool[])
        n210 = call "Verdichternamen.vi"("Array"=w119) -> ("Dynamic Data"=w375:dynamicdata)  [unwired: 10 in]
        n211 = Seconds To Date/Time(time stamp (now)=w377) -> (date time rec=w321:T15)  [unwired: 1 in]
        n212 = Seconds To Date/Time(time stamp (now)=w381) -> (date time rec=w390:T15)  [unwired: 1 in]
        n213 = Unbundle By Name(w390) -> ("second"=w389:i32, "minute"=w388:i32, "hour"=w382:i32)
        n214 = Unbundle By Name(w321) -> ("second"=w392:i32, "minute"=w391:i32, "hour"=w379:i32)
        n215 = Bundle("second"=w392, "minute"=w391, "hour"=w379) -> (→"Verdichteraktivität":cluster{"second":i32, "minute":i32, "hour":i32})  [unwired: 1 in]
        n216 = Bundle("second"=w389, "minute"=w388, "hour"=w382) -> (→"Betriebszeit":cluster{"second":i32, "minute":i32, "hour":i32})  [unwired: 1 in]
        n217 = Merge Signals(w145, w144, w264, w375) -> (w283:dynamicdata)
        n218 = flat-sequence {
          tunnel: [w485] -> w402
          tunnel: [w484] -> w401
          tunnel: w301 -> [w483]
          tunnel: w300 -> [w482]
          tunnel: [w480] -> w297
          tunnel: "Identität!" -> [w479]
          tunnel: "Dateiname!" -> [w478]
          tunnel: "Speichern" -> [w477]
          tunnel: "tag" -> [w476]
          tunnel: w402 -> [w583]
          tunnel: w401 -> [w582]
          tunnel: [w578] -> w304
          tunnel: [w580] -> w303
          tunnel: w302 -> [w579]
          frame #0 {
            n219 = Index Array(array=w482) -> (element=w481:timestamp)  [unwired: 1 in]
            n220 = event shown="[1] \"Speichern\": Value Change" {
              selector: _ -> [_ _ _]
              dyn-events: _ -> [_ _ _]
              timeout: 5 -> [_ _ _]
              tunnel: [_ w495 _] -> w485
              tunnel: w483 -> [_ w490 _]
              tunnel: ["" w494 ""] -> w484
              tunnel: w481 -> [_ w493 w564]
              tunnel: [_ _ w562] -> w480
              tunnel: w479 -> [_ w492 _]
              tunnel: w478 -> [_ w491 _]
              tunnel: w477 -> [_ w489 _]
              tunnel: w476 -> [_ w488 _]
              event Timeout {
                n221 = event-data() -> ()  [unwired: 1 in, 1 out]
              }
              event "Speichern": Value Change {
                n222 = event-data() -> ()  [unwired: 1 in, 1 out]
                n223 = case shown="True" w489 {
                  tunnel: [w527 _] -> w495
                  tunnel: [w522 _] -> w494
                  tunnel: w493 -> [w514 _]
                  tunnel: w492 -> [w498 _]
                  tunnel: w491 -> [w510 _]
                  tunnel: w490 -> [w509 _]
                  tunnel: w488 -> [w497 _]
                  frame False {
                    w501 = "\r"
                    n224 = property on="Dateiname!" class="Str"("DisabledEnum"=T4."Disabled and Grayed Out" ("Disabled")) -> ()  [unwired: 2 in, 2 out]
                    n225 = for {
                      N: 1 -> [_]
                      tunnel: ["Zeit"] -> w507 mode=indexing
                      tunnel: ["Kommentar"] -> w503 mode=indexing
                    }
                    n226 = Format Date/Time String(time format string (%c)="%d-%m-%Y_%H.%M ", seconds (now)=w514) -> (date/time string=w515:string)  [unwired: 1 in]
                    n227 = Concatenate Strings(w498, "\\", w515, w510, ".lvm" ("string")) -> (w517:string)
                    n228 = Insert Into Array(array=w509, index (row)=0, new element=w507) -> (w505:string[][])  [unwired: 1 in]
                    n229 = Build Path(base path=path "\\\\pcift88\\Studenten/HT-Waermepumpe/Messdaten" ("file path (dialog if empty)"), name or relative path=w517) -> (appended path=w512:path)
                    n230 = Concatenate Strings(w498, "\t", "tag: " ("string"), w497) -> (w496:string)
                    n231 = Insert Into Array(array=w505, new element=w503) -> (w504:string[][])  [unwired: 2 in]
                    n232 = Open/Create/Replace File(file path (use dialog)=w512, operation (0:open)=T11."replace or create with confirmation") -> (refnum out=→"refnum out":refnum<file>, error out=w527:errorcluster)  [unwired: 4 in, 1 out]
                    n233 = Transpose 2D Array(2D array=w504) -> (transposed array=w525:string[][])
                    n234 = Format Date/Time String(seconds (now)=w514) -> (date/time string=w524:string)  [unwired: 2 in]
                    n235 = Strip Path(path=w512) -> (name=w511:string)  [unwired: 1 out]
                    n236 = Array To Spreadsheet String(array=w525, 3:"%s" ("format string")) -> (spreadsheet string=w523:string)  [unwired: 1 in]
                    n237 = Concatenate Strings(w496, w501, w501, w511, w501, w501, w524, w501, w501, w523, w501, w501) -> (w522:string)
                  }
                  frame True {
                    n238 = local read "refnum out"() -> (w531:refnum<file>)
                    n239 = property on="Dateiname!" class="Str"("DisabledEnum"=T4."Enabled" ("Disabled")) -> ()  [unwired: 2 in, 2 out]
                    n240 = Close File(refnum=w531) -> ()  [unwired: 1 in, 2 out]
                  }
                }
              }
              event "Comment": Value Change {
                # "Umlaute + ß ersetzen, quick&dirty 4.1.2016"
                n241 = event-data() -> ()  [unwired: 1 in, 1 out]
                n242 = flat-sequence {
                  tunnel: ["Kommentar"] -> w532
                  tunnel: w564 -> [w568]
                  frame #0 {
                    w570 = "\r"
                    n243 = local read "Historie"() -> (w572:string)
                    n244 = Get Date/Time String(seconds (now)=w568, want seconds? (F)=TRUE) -> (time string=w571:string)  [unwired: 1 in, 1 out]
                    n245 = Concatenate Strings(w572, w571, " -> ", "Kommentar", w570, w570) -> (→"Historie":string)
                  }
                  frame #1 {
                    n246 = local write "Kommentar"("") -> ()
                  }
                }
                n247 = Search and Replace String(replace all?=TRUE, input string=w532, search string="ä", replace string="ae") -> (result string=w554:string)  [unwired: 4 in, 3 out]
                n248 = Search and Replace String(replace all?=TRUE, input string=w554, search string="ü", replace string="ue") -> (result string=w553:string)  [unwired: 4 in, 3 out]
                n249 = Search and Replace String(replace all?=TRUE, input string=w553, search string="ö", replace string="oe") -> (result string=w552:string)  [unwired: 4 in, 3 out]
                n250 = Search and Replace String(replace all?=TRUE, input string=w552, search string="ß", replace string="ss") -> (result string=w533:string)  [unwired: 4 in, 3 out]
                n251 = Search and Replace String(replace all?=TRUE, input string=w533, search string="Ä", replace string="Ae") -> (result string=w542:string)  [unwired: 4 in, 3 out]
                n252 = Search and Replace String(replace all?=TRUE, input string=w542, search string="Ü", replace string="Ue") -> (result string=w541:string)  [unwired: 4 in, 3 out]
                n253 = Search and Replace String(replace all?=TRUE, input string=w541, search string="Ö", replace string="Oe") -> (result string=w534:string)  [unwired: 4 in, 3 out]
                n254 = for {
                  N: 1 -> [_]
                  tunnel: [w565] -> w562 mode=indexing
                  tunnel: w534 -> [w565]
                }
              }
            }
          }
          frame #1 {
            n255 = local read "refnum out"() -> (w575:refnum<file>)
            n256 = Concatenate Strings(w582, w579) -> (w581:string)
            n257 = Not A Number/Path/Refnum?(number/path/refnum=w575) -> (NaN/Path/Refnum?=w576:bool)
            n258 = Set File Position(refnum=w575, from (0:start)=enum16{"start", "end", "current"}."end", error in=w583) -> (refnum out=w584:refnum<file>, error out=w585:errorcluster)  [unwired: 1 in]
            n259 = Not(x=w576) -> (.not. x?=→"Speichert!":bool)
            n260 = Write to Text File(file (use dialog)=w584, text=w581, error in=w585) -> (refnum out=w578:refnum<file>, error out=w580:errorcluster)  [unwired: 1 in, 1 out]
          }
        }
        n261 = Empty String/Path?(string/path="Identität!") -> (empty?=w295:bool)
        n262 = Empty String/Path?(string/path="Dateiname!") -> (empty?=w294:bool)
        n263 = Or(x=w295, y=w294) -> (x .or. y?=w291:bool)
        n264 = call "Protokollordnung"("Signals"=w283) -> ("Signal Out"=w309:dynamicdata)  [unwired: 9 in, 1 out]
        n265 = Boolean To (0,1)(Boolean=w291) -> (0, 1=w292:i16)
        n266 = expression code="x*2"(w292) -> (w293:i16)
        n267 = property on="Speichern" class="Bool (strict)"("DisabledEnum"=w293) -> ()  [unwired: 2 in, 2 out]
        n268 = call "Convert from Dynamic Data"("Dynamic Data Type"=w309) -> ("Array of Waveform"=w310:waveform(dbl)[])  [unwired: 3 in]
        n269 = Array Size(array=w310) -> (size(s)=w287:i32)
        n270 = Concatenate Strings("%" ("string"), "." ("string"), ";%g" ("string")) -> (w312:string)
        n271 = Initialize Array(w312, w287) -> (w311:string[])
        n272 = for {
          tunnel: w310 -> [w589] mode=indexing
          tunnel: [w596] -> w307 mode=indexing
          tunnel: w311 -> [w594] mode=indexing
          tunnel: [w588] -> w301 mode=indexing
          tunnel: [w590] -> w300 mode=indexing
          tunnel: [w591] -> w306 mode=indexing
          n273 = Unbundle By Name(w589) -> ("Y"=w595:dbl[], "t0"=w587:timestamp)
          n274 = Get Waveform Attribute(5:w587, 6:"NI_ExpTimeStamp", 7:w589) -> (1:w590:timestamp)  [unwired: 1 in, 3 out]
          n275 = for {
            tunnel: w595 -> [w603] mode=indexing
            tunnel: [w602] -> w596 mode=indexing
            tunnel: w594 -> [w601]
            tunnel: w589 -> [w600]
            tunnel: [w599] -> w588 mode=indexing
            n276 = Format Into String(format string=w601, w603) -> (resulting string=w602:string)  [unwired: 2 in, 1 out]
            n277 = Get Waveform Attribute(5:"", 6:"NI_ChannelName", 7:w600) -> (1:w599:string)  [unwired: 1 in, 3 out]
          }
          n278 = Format Date/Time String(time format string (%c)="%H.%M.%S", seconds (now)=w590) -> (date/time string=w591:string)  [unwired: 1 in]
        }
        n279 = Insert Into Array(array=w307, index (row)=0, new element=w306) -> (w298:string[][])  [unwired: 1 in]
        n280 = Increment(x=w287) -> (x+1=w288:i32)
        n281 = Insert Into Array(array=w298, index (row)=w288, new element=w297) -> (w299:string[][])  [unwired: 1 in]
        n282 = Transpose 2D Array(2D array=w299) -> (transposed array=w296:string[][])
        n283 = Array To Spreadsheet String(array=w296, 3:"%s" ("format string")) -> (spreadsheet string=w302:string)  [unwired: 1 in]
      }
      frame #2 {
        n284 = Tick Count (ms)() -> (millisecond timer value=w721:u32)
        n285 = Subtract(x=w721, y=w720) -> (x-y=w719:u32)
        n286 = Divide(x=w719, y=1000.0) -> (x/y=→"Schleifendauer":dbl)
      }
    }
  }
  n287 = call <vilib>:"DAQmx Clear Task.vi"("task in"=w6, "error in"=w4) -> ()  [unwired: 13 in, 1 out]
  n288 = call <vilib>:"DAQmx Clear Task.vi"("task in"=w5, "error in"=w3) -> ()  [unwired: 13 in, 1 out]
  n289 = Close File(refnum=w31, error in=w30) -> (error out=w34:errorcluster)  [unwired: 1 out]
  n290 = call <vilib>:"General Error Handler.vi"("error in (no error)"=w34, "[exception action] (none:0)"=1 ("[exception code]"), "[exception code]"=1) -> ()  [unwired: 8 in, 5 out]
